vi "UpTempServer.vi"() -> ()   [LabVIEW 2024]
panel:
  in  "Sampling Period":i64=1000
  out "TLUP_Temperatures":waveform(dbl)[](array[waveform])
  out "Waveform Chart":waveform(dbl)[](graph)
  in  "stop":bool
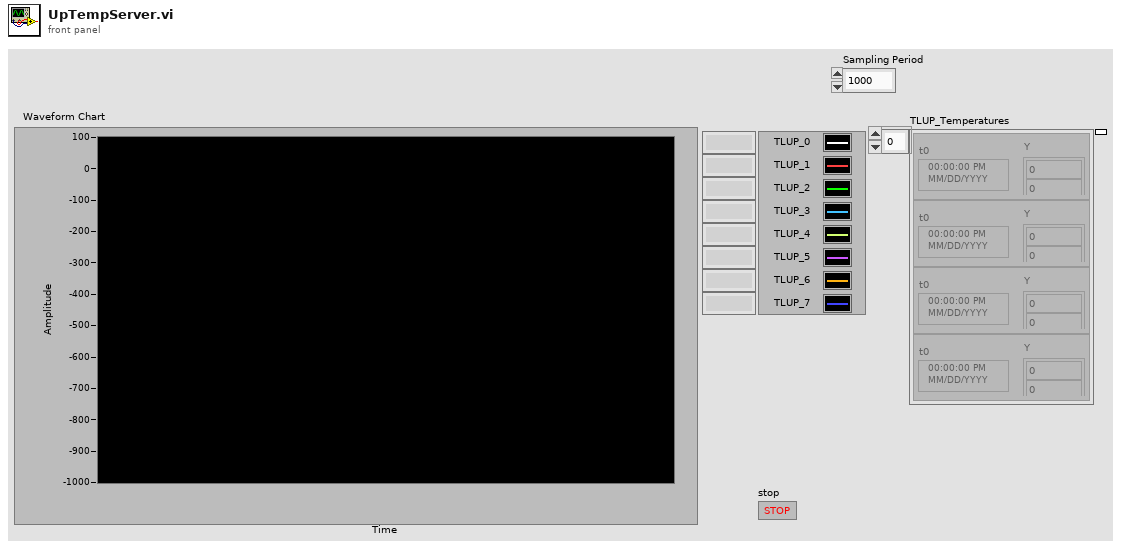
[diagram p1: front panel]
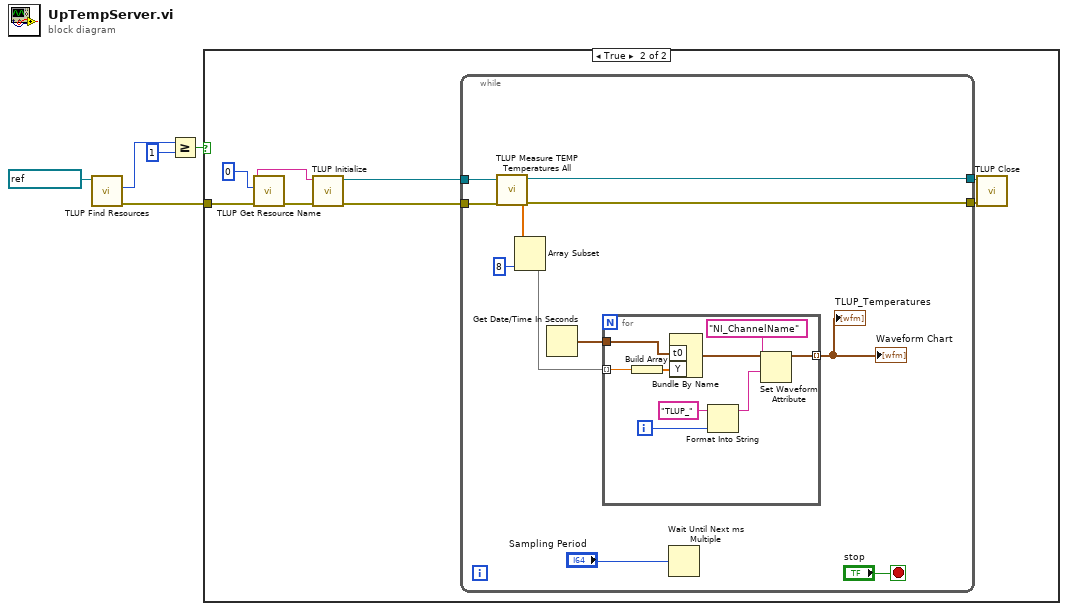
[diagram p0: block diagram]
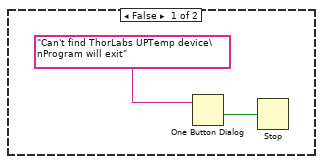
[diagram p2: hidden frame]
diagram:
  n1 = call <instrlib>:"TLUP Find Resources.vi"("instrument handle"=refnum<visa-resource-name> "UpTemp" ("resource name")) -> ("error out"=w4:errorcluster, "Resource Count"=w2:u32)  [unwired: 8 in, 1 out]
  n2 = Greater Or Equal?(x=w2, y=u32 1) -> (x >= y?=w3:bool)
  n3 = case shown="True" w3 {
    tunnel: w4 -> [_ w11]
    frame False {
      n4 = One Button Dialog(message="Can't find ThorLabs UPTemp device\nProgram will exit") -> (true=w6:bool)  [unwired: 1 in]
      n5 = Stop(stop? (T)=w6) -> ()
    }
    frame True {
      n6 = call <instrlib>:"TLUP Get Resource Name.vi"("error in (no error)"=w11, "Index (0)"=u32 0) -> ("error out"=w9:errorcluster, "Resource Name"=w8:string)  [unwired: 7 in, 1 out]
      n7 = call <instrlib>:"TLUP Initialize.vi"("error in (no error)"=w9, "resource name"=w8) -> ("error out"=w14:errorcluster, "instrument handle out"=w15:refnum<visa-resource-name>)  [unwired: 8 in]
      n8 = while {
        tunnel: w15 -> [w26]
        tunnel: w14 -> [w25]
        tunnel: [w24] -> w12
        tunnel: [w23] -> w13
        stop <- "stop" stop-if-true
        n9 = call <instrlib>:"TLUP Measure TEMP Temperatures All.vi"("error in (no error)"=w25, "instrument handle"=w26) -> ("error out"=w23:errorcluster, "Measurement Values (0.0)"=w21:dbl[], "instrument handle out"=w24:refnum<visa-resource-name>)  [unwired: 6 in, 1 out]
        n10 = Array Subset(array=w21, length=8) -> (w18:dbl[])  [unwired: 1 in]
        n11 = Get Date/Time In Seconds() -> (seconds since 1Jan1904=w20:timestamp)
        n12 = for {
          tunnel: w18 -> [w34] mode=indexing
          tunnel: w20 -> [w33]
          tunnel: [w31] -> w19 mode=indexing
          i -> [w28]
          n13 = Build Array(w34) -> (w35:dbl[])
          n14 = Bundle By Name("t0"=w33, "Y"=w35) -> (w32:waveform(dbl))  [unwired: 1 in]
          n15 = Format Into String(initial string="TLUP_", w28) -> (resulting string=w27:string)  [unwired: 2 in, 1 out]
          n16 = Set Waveform Attribute(5:w27, 6:"NI_ChannelName" ("name"), 7:w32) -> (3:w31:waveform(dbl))  [unwired: 1 in, 2 out]
        }
        "Waveform Chart" <- w19
        "TLUP_Temperatures" <- w19
        n17 = Wait Until Next ms Multiple(millisecond multiple="Sampling Period") -> ()  [unwired: 1 out]
      }
      n18 = call <instrlib>:"TLUP Close.vi"("error in (no error)"=w13, "instrument handle"=w12) -> ()  [unwired: 9 in, 1 out]
    }
  }
